vi "Signal All VIs to Stop.vi"(8 "error in (no error)":errorcluster) -> (0 "error out":errorcluster)   [LabVIEW 2017]
uses:
  General Globals.vi
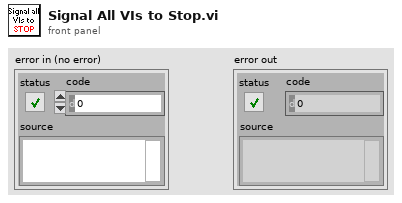
[diagram p1: front panel]
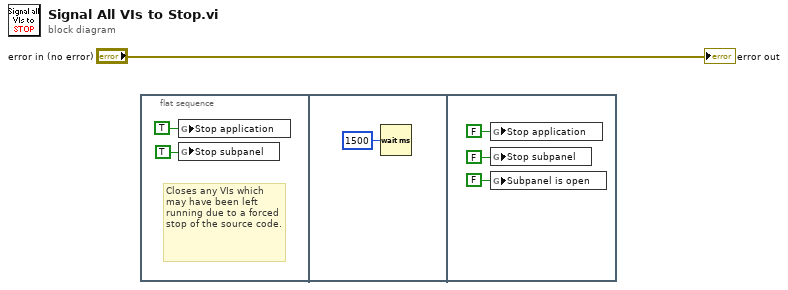
[diagram p0: block diagram]
diagram:
  n1 = flat-sequence {
    frame #0 {
      # "Closes any VIs which may have been left running due to a forced stop of the source code."
      n2 = global write "General Globals.vi" "Stop application"(TRUE ("Stop application")) -> ()
      n3 = global write "General Globals.vi" "Stop subpanel"(TRUE ("Stop subpanel")) -> ()
    }
    frame #1 {
      n4 = Wait (ms)(milliseconds to wait=u32 1500) -> ()  [unwired: 1 out]
    }
    frame #2 {
      n5 = global write "General Globals.vi" "Stop application"(FALSE ("Stop application")) -> ()
      n6 = global write "General Globals.vi" "Stop subpanel"(FALSE ("Stop subpanel")) -> ()
      n7 = global write "General Globals.vi" "Subpanel is open"(FALSE ("Subpanel is open")) -> ()
    }
  }
  "error out" <- "error in (no error)"
